vi "REACTOR_MODO MANUAL.vi"(5 "Modulo":u32, 7 "Secuencia":string[](array[string]), 8 "error in (no error)":errorcluster, 9 "ALICATS":T4=[["3", "NO", "M0000013", "Air", "10", "ln/mn", "0", "0"], ["4", "NO", "M0000014", "Air", "10", "ln/mn", "0", "0"], ["5", "NO", "M0000015", "Air", "10", "ln/mn", "0", "0"], ["6", "NO", "M0000016", "Air", "10", "ln/mn", "0", "0"], ["7", "NO", "M0000017", "Air", "10", "ln/mn", "0", "0"], ["8", "NO", "M0000018", "Air", "10", "ln/mn", "0", "0"]], 11 "Comms":T5={"Alicats"="ASRL6::INSTR", "Alic"=FALSE, "eValve"="ASRL6::INSTR", "eval"=FALSE, "Eurotherm"="ASRL6::INSTR", "euro"=FALSE, "Cell GAS"="ASRL6::INSTR", "cgas"=FALSE, "Cell H2S"="ASRL6::INSTR", "ch2s"=FALSE}) -> (0 "error out":errorcluster)   [LabVIEW 2017]
uses:
  REACTOR_DATOS.ctl
  REACTOR_COMUNICACIONES.ctl
  SERIAL ALICATS/__s_TablaAlicats.ctl
  SERIAL ALICATS/__Alicat SD_ReadingCluster.ctl
  EUROTHERM/TEG P116x2.ctl
  EUROTHERM/2xP116.ctl
  DISPLAY/Data Type.ctl
  DISPLAY/Display_Command Control.ctl
  REACTOR_MODO MANUAL.ctl
  FILE/File_Module Control.ctl
  TIMING/Timing_Module Control.ctl
  EUROTHERM/Eurotherm_New_Module.ctl
  REACTOR_CHANGE.ctl
  SERIAL RASP_PICO VALVE/kissia_rasPico Module.ctl
  REACTOR_GLOBALES.vi
panel:
  out "Fecha":string caption="asd"
  out "ERRORES_T":i32=5 caption="Elapsed Time (s)"
  out "VALVE":bool
  out "P116x2":T1
  out "ParsedReadingArray":T3[](array[typedef]) {"Total" format="%.2f"; "SetPoint" format="%.2f"; "Mass" format="%.2f"; "Volumetric" format="%.2f"; "Temperature" format="%.2f"; "Pressure" format="%.2f"}
  out "LEER ?":bool=TRUE
  in  "T.Wait Stability":bool
  in  "Mide Alicats":bool=TRUE
  in  "Mide Temperaturas":bool=TRUE
  in  "Muestreo(s)":dbl=1.0
  out "TIEMPO (m)":dbl
  out "Timestring":string
  out "idxModulo":u32
  out "Max_t(s)":dbl format="%.1f"
  out "Delta t(s)":dbl format="%.1f"
  out "Delta T(C)":dbl format="%.1f"
  out "TStable":bool
  out "Datos":T6 {"a FSET4" format="%.2g"; "a FSET3" format="%.2g"; "a FSET2" format="%.2g"; "a FSET1" format="%.2g"; "a FLUJO4" format="%.2g"; "a FLUJO2" format="%.2g"; "a FLUJO1" format="%.2g"; "a FLUJO3" format="%.2g"; "eVAL_5" format="%.2g"; "TEMP_TH" format="%.2g"; "SET_TH" format="%.2g"; "TEMP_TC" format="%.2g"; "SET_TC" format="%.2g"; "TIEMPO" format="%.2g"}
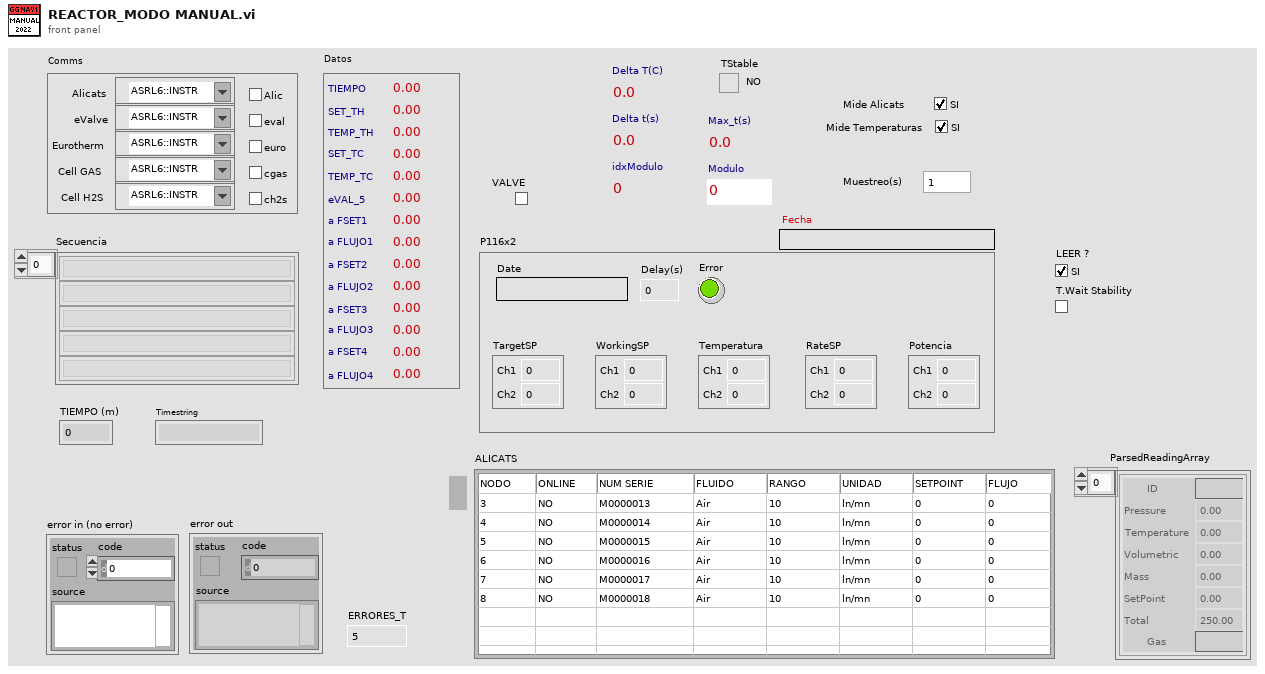
[diagram p1: front panel]
types:
  T1 = typedef "TEG P116x2.ctl" = cluster{"TargetSP":T2, "WorkingSP":T2, "Temperatura":T2, "Error":bool, "Date":string, "Delay(s)":dbl, "RateSP":T2, "Potencia":T2}
  T2 = typedef "2xP116.ctl" = cluster{"Ch1":dbl, "Ch2":dbl}
  T3 = typedef "__Alicat SD_ReadingCluster.ctl" = cluster{"ID":string, "Pressure":sgl, "Temperature":sgl, "Volumetric":sgl, "Mass":sgl, "SetPoint":sgl, "Gas":string, "Total":sgl}
  T4 = typedef "__s_TablaAlicats.ctl" = string[][]
  T5 = typedef "REACTOR_COMUNICACIONES.ctl" = cluster{"Alicats":refnum<visa-resource-name>, "Alic":bool, "eValve":refnum<visa-resource-name>, "eval":bool, "Eurotherm":refnum<visa-resource-name>, "euro":bool, "Cell GAS":refnum<visa-resource-name>, "cgas":bool, "Cell H2S":refnum<visa-resource-name>, "ch2s":bool}
  T6 = typedef "REACTOR_DATOS.ctl" = cluster{"TIEMPO":dbl, "SET_TH":dbl, "TEMP_TH":dbl, "SET_TC":dbl, "TEMP_TC":dbl, "eVAL_5":dbl, "a FSET1":dbl, "a FLUJO1":dbl, "a FSET2":dbl, "a FLUJO2":dbl, "a FSET3":dbl, "a FLUJO3":dbl, "a FSET4":dbl, "a FLUJO4":dbl}
  T7 = typedef "REACTOR_MODO MANUAL.ctl" = enum16{"INICIALIZAR", "LEER TIEMPO", "LEER TEMPERATURAS", "LEER ALICATS", "TEMPERATURAS ESTABLES ?", "GUARDAR DATOS", "WAIT NEXT", "HAY CAMBIOS ?", "FINALIZAR"}
  T8 = typedef "Data Type.ctl" = enum16{"Init FP", "En/Dis FP Ctls", "Update FP", "Upd Status", "Upd Seq"}
  T9 = typedef "Display_Command Control.ctl" = enum16{"Initialize", "Generate Event", "Shutdown"}
  T10 = typedef "File_Module Control.ctl" = enum16{"Initialize", "Save Head", "Save Data", "Shutdown"}
  T11 = typedef "Timing_Module Control.ctl" = enum16{"Initialize Time", "Check Time"}
  T12 = typedef "Eurotherm_New_Module.ctl" = enum16{"Initialize", "Write SP", "Read SP+PV", "Write Rate", "Set P", "Set I", "Set D", "Shutdown"}
  T13 = typedef "REACTOR_CHANGE.ctl" = enum16{"Default", "Continue", "Change Alicats", "Change Valve", "Change Calor", "Change Frio"}
  T14 = typedef "kissia_rasPico Module.ctl" = enum16{"Initialize", "Read Data", "Write Data", "Enable", "Disable", "Shutdown"}
  T15 = enum16{"Add 1", "Add 2", "Add 10", "Add 11", "Add 12", "Add 13"}[]
  T16 = cluster{"processVal":dbl, "targetSP":dbl, "workingSP":dbl, "workingOut":dbl}
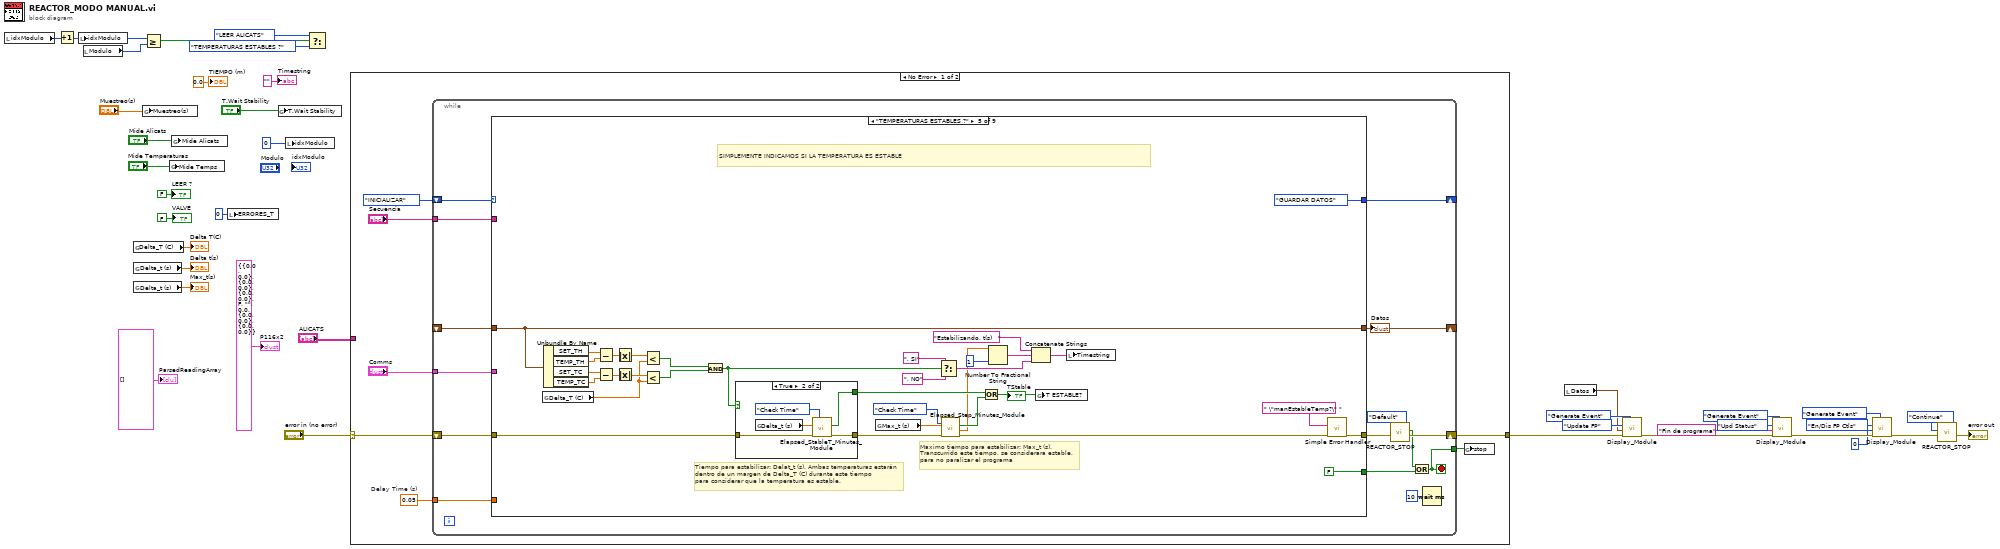
[diagram p0: block diagram]
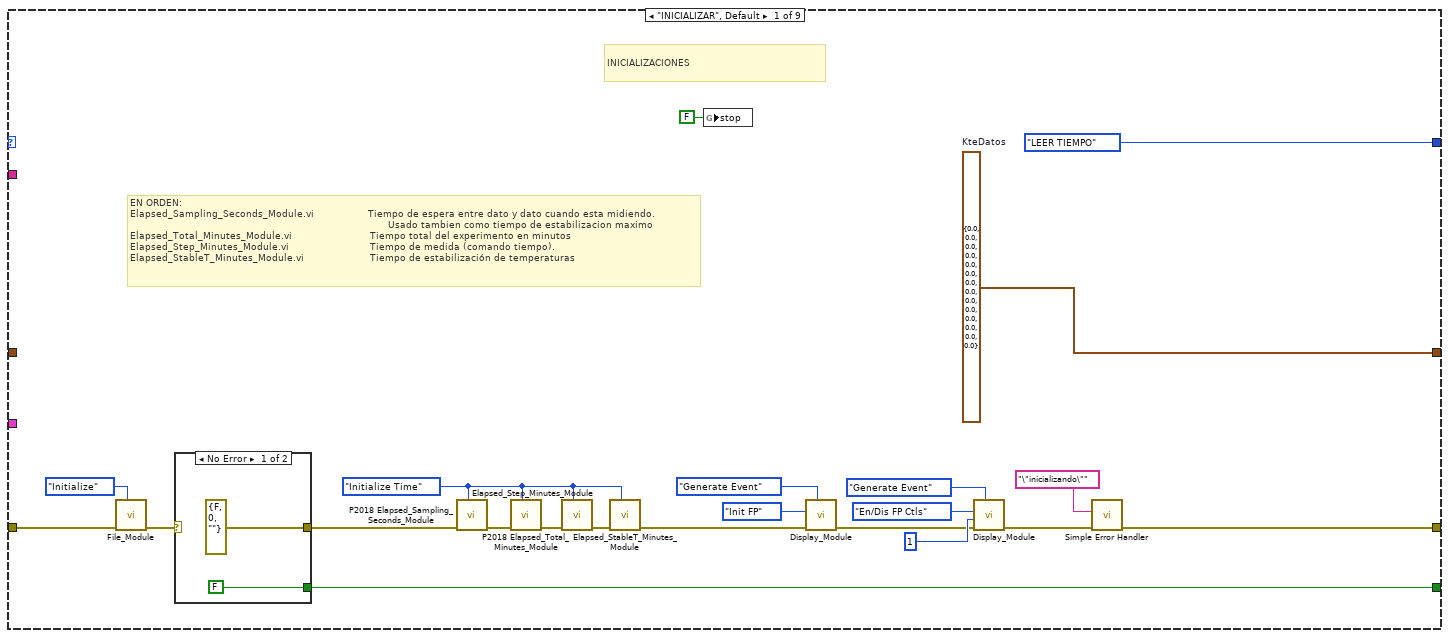
[diagram p2: hidden frame]
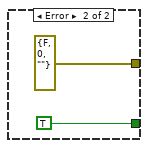
[diagram p3: hidden frame]
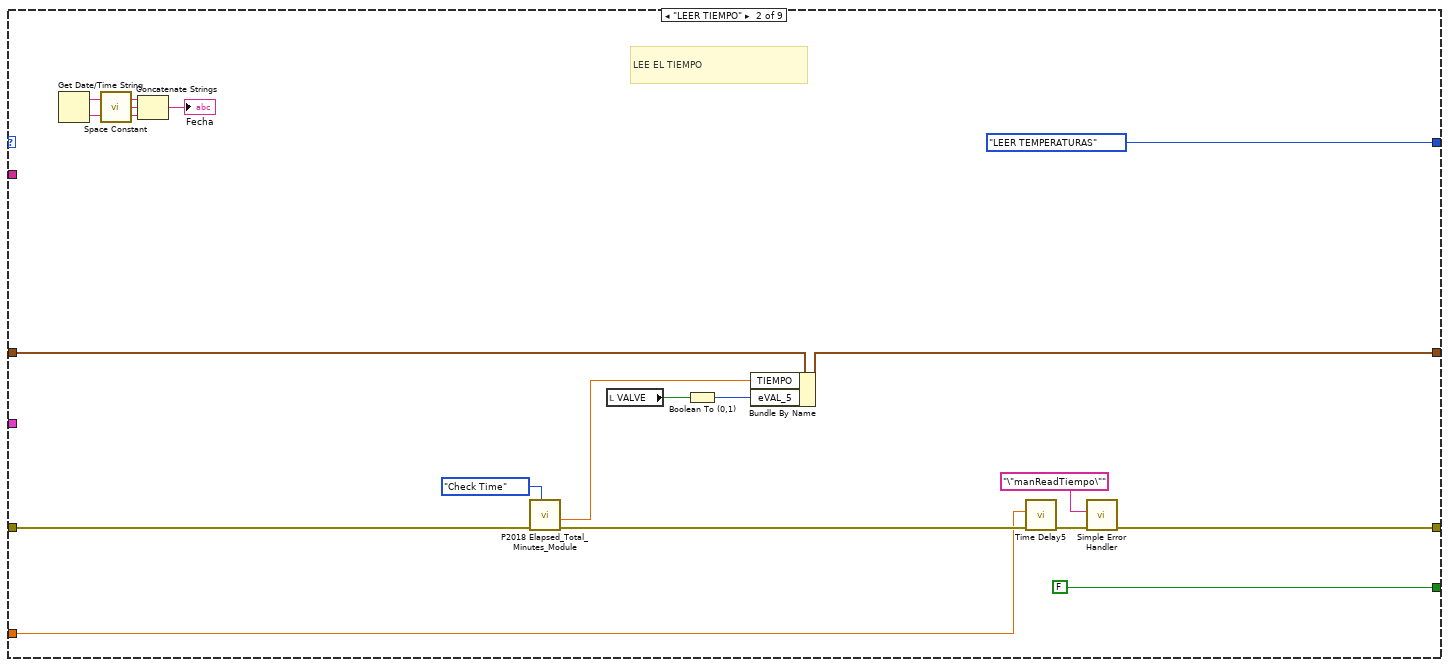
[diagram p4: hidden frame]
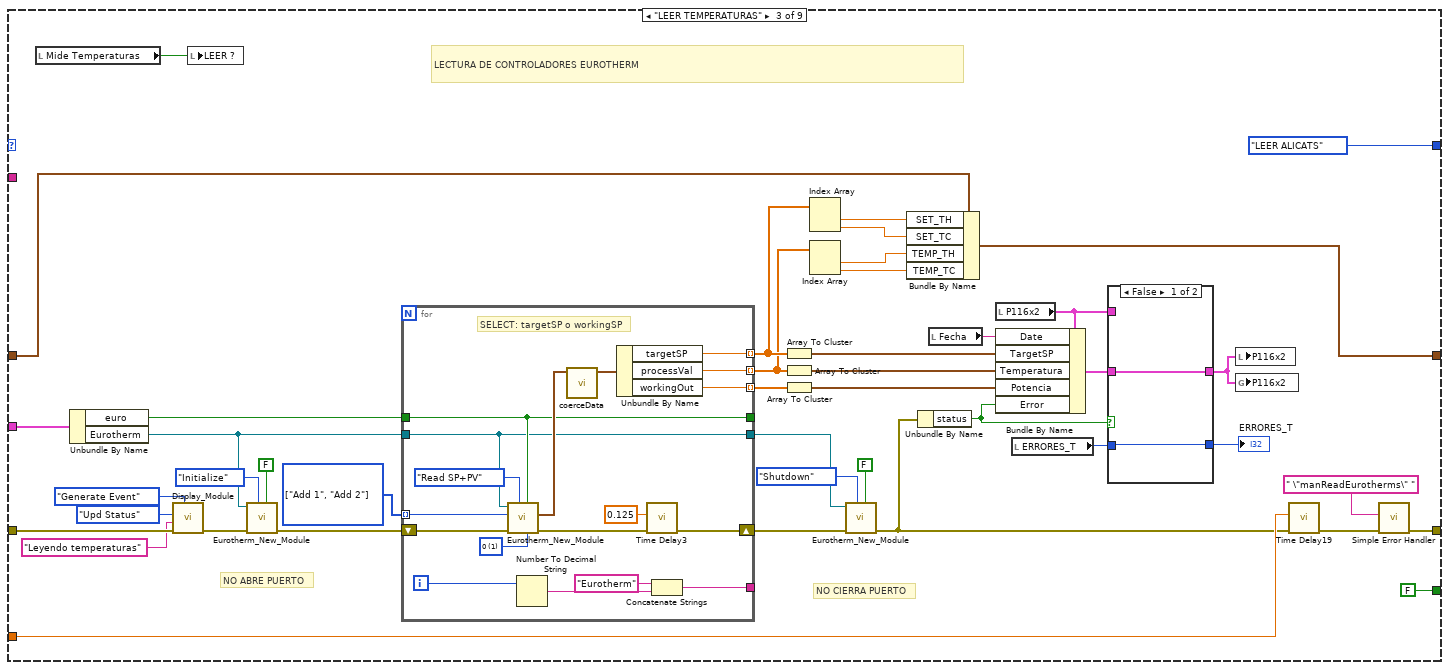
[diagram p5: hidden frame]
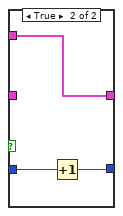
[diagram p6: hidden frame]
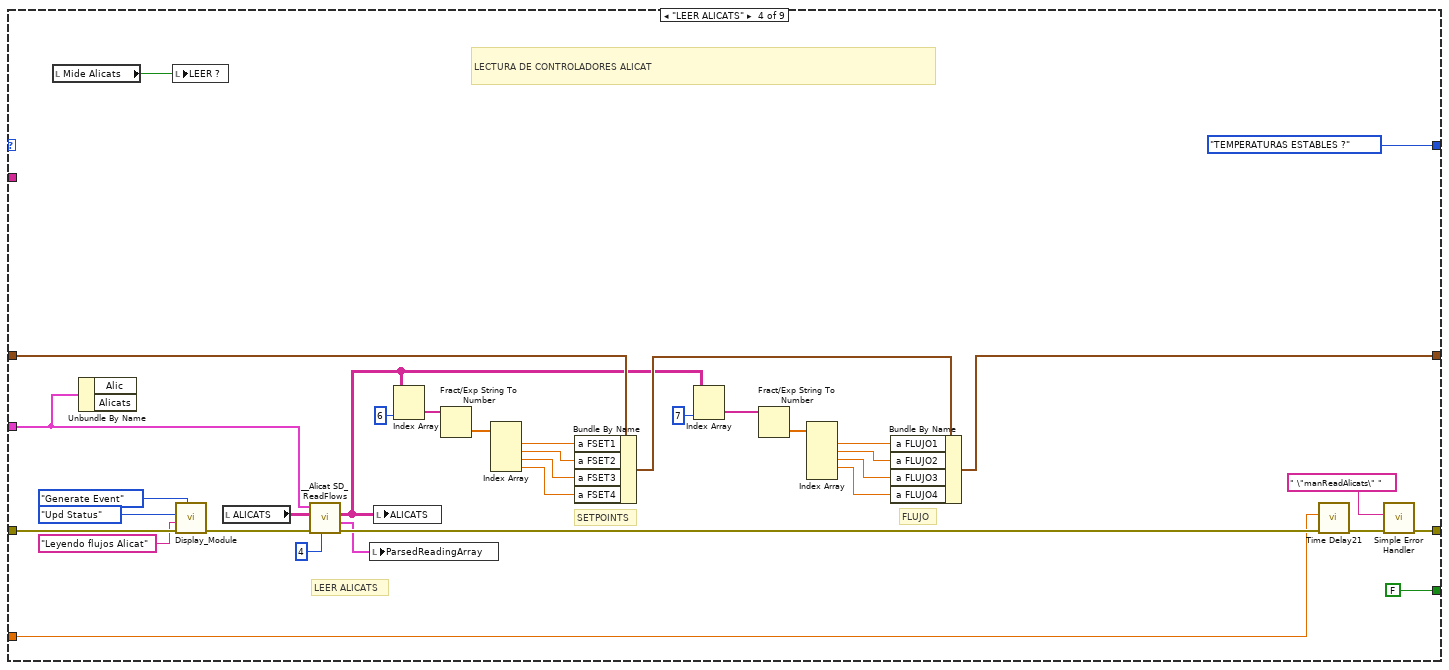
[diagram p7: hidden frame]
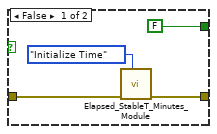
[diagram p8: hidden frame]
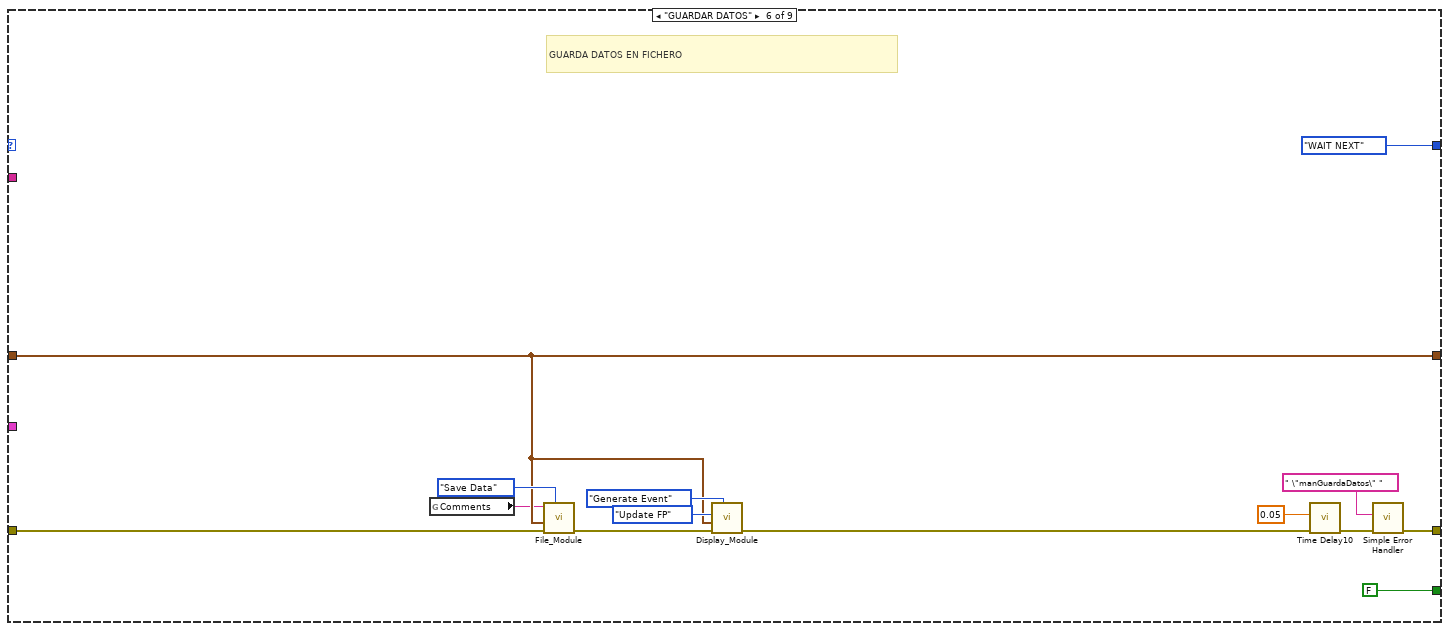
[diagram p9: hidden frame]
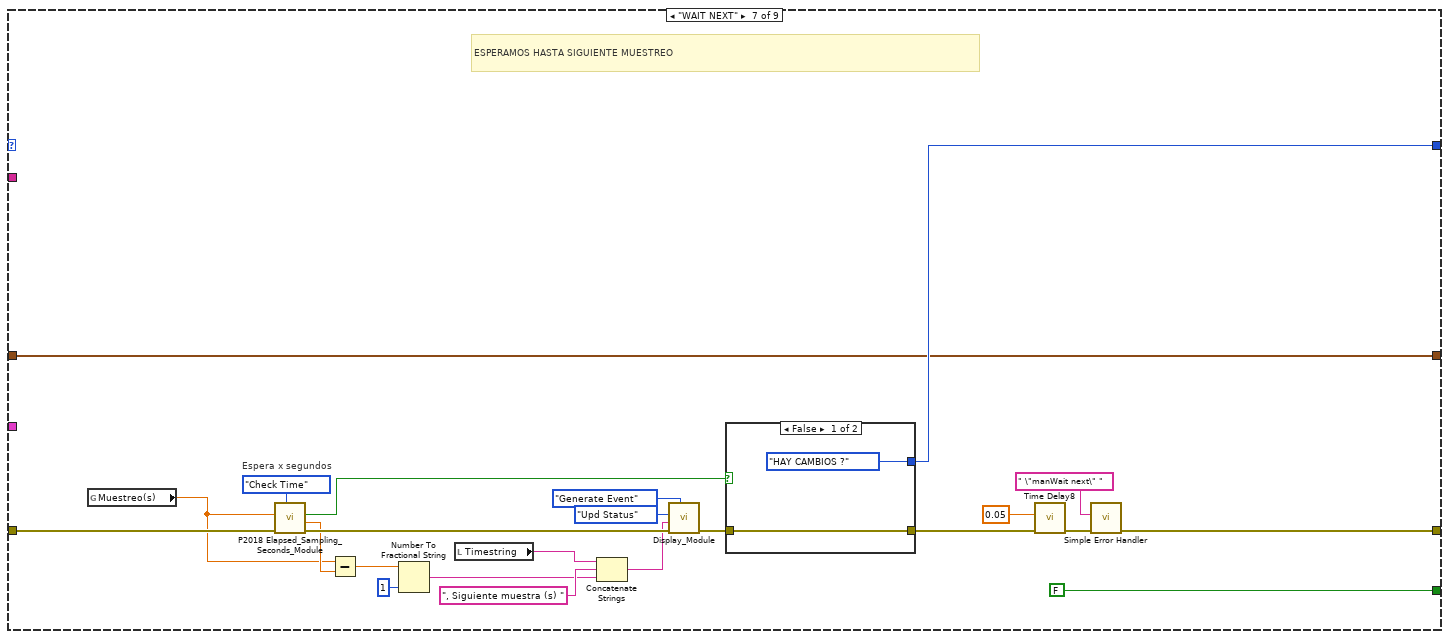
[diagram p10: hidden frame]
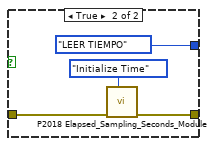
[diagram p11: hidden frame]
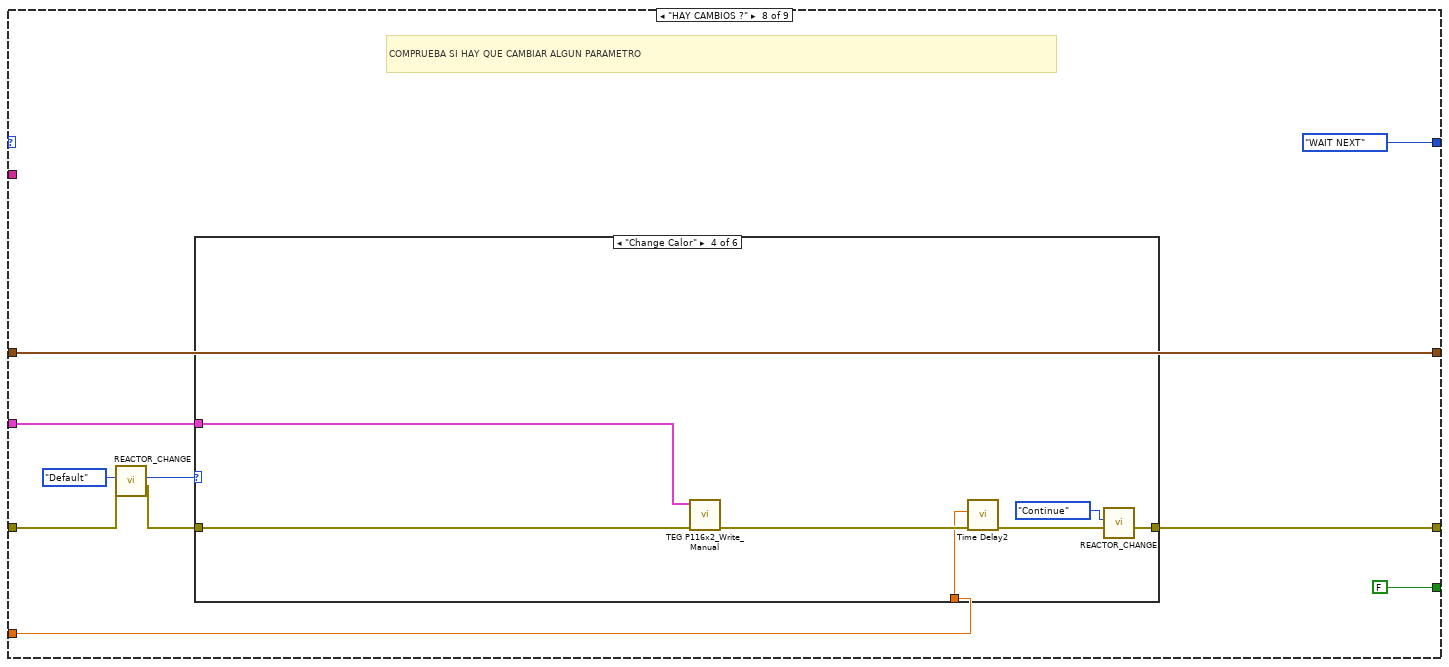
[diagram p12: hidden frame]
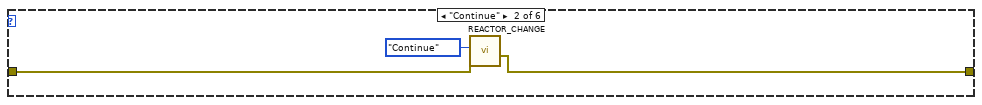
[diagram p14: hidden frame]
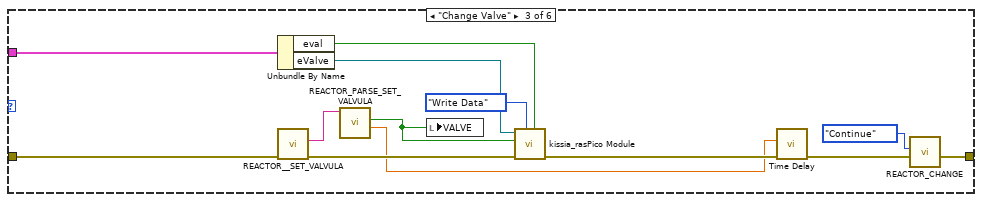
[diagram p15: hidden frame]
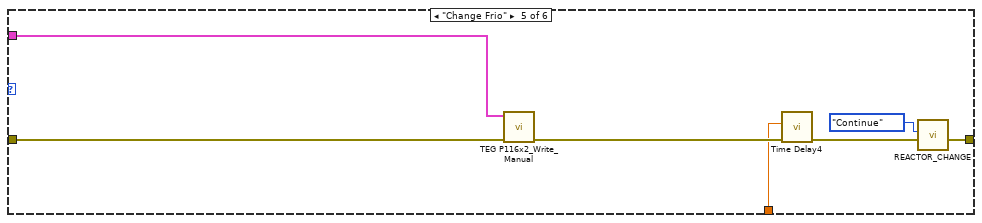
[diagram p16: hidden frame]
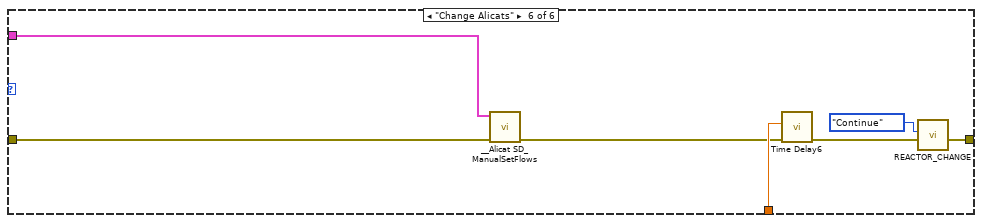
[diagram p17: hidden frame]
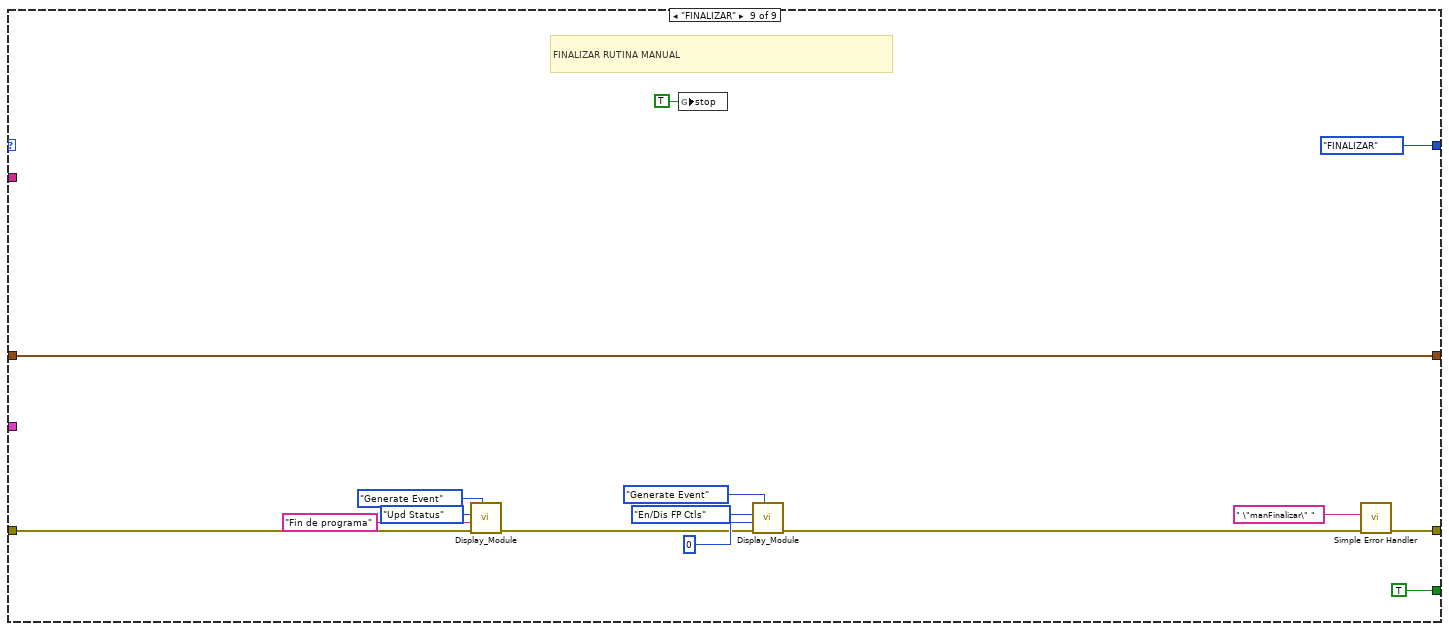
[diagram p18: hidden frame]
diagram:
  n1 = local read "idxModulo"() -> (w3:u32)
  n2 = Increment(x=w3) -> (x+1=w4:u32)
  n3 = local write "idxModulo"(w4) -> ()
  n4 = local read "Modulo"() -> (w6:u32)
  n5 = global read "REACTOR_GLOBALES.vi" "Delta_T (C)"() -> (→"Delta T(C)":dbl)
  n6 = global read "REACTOR_GLOBALES.vi" "Delta_t (s)"() -> (→"Delta t(s)":dbl)
  n7 = global read "REACTOR_GLOBALES.vi" "Delta_t (s)"() -> (→"Max_t(s)":dbl)
  n8 = global write "REACTOR_GLOBALES.vi" "Muestreo(s)"("Muestreo(s)") -> ()
  n9 = Greater Or Equal?(x=w4, y=w6) -> (x >= y?=w5:bool)
  n10 = global write "REACTOR_GLOBALES.vi" "Mide Temps"("Mide Temperaturas") -> ()
  n11 = global write "REACTOR_GLOBALES.vi" "Mide Alicats"("Mide Alicats") -> ()
  n12 = local write "ERRORES_T"(0 ("ERRORES_T")) -> ()
  n13 = global write "REACTOR_GLOBALES.vi" "T.Wait Stability"("T.Wait Stability") -> ()
  n14 = local write "idxModulo"(u32 0 ("MedidaModulo")) -> ()
  n15 = Select(t=REACTOR_MODO_MANUAL."LEER ALICATS" ("Command"), s=w5, f=REACTOR_MODO_MANUAL."TEMPERATURAS ESTABLES ?" ("Command")) -> ()  [unwired: 1 out]
  n16 = case shown="No Error" "error in (no error)" {
    selector: "error in (no error)" -> [w45 w354]
    tunnel: [w44 w354] -> w8
    tunnel: "ALICATS" -> [_ _]
    frame No Error {
      w40 = 0.05  # Delay Time (s)
      n17 = while {
        shift-right: [w56] -> _
        shift-left: REACTOR_MODO_MANUAL."INICIALIZAR" ("Command") -> [w57]
        shift-right: [w49] -> w44
        shift-left: w45 -> [w58]
        shift-right: [w53] -> _
        shift-left: _ -> [w55]
        tunnel: "Secuencia" -> [w54]
        tunnel: "Comms" -> [w52]
        tunnel: w40 -> [w51]
        tunnel: [w46] -> w39
        stop <- w46 stop-if-true
        n18 = case shown="\"TEMPERATURAS ESTABLES ?\"" w57 {
          tunnel: [w71 FALSE FALSE FALSE FALSE FALSE FALSE FALSE TRUE] -> w59
          tunnel: w58 -> [w81 w101 w144 w204 w208 w261 w278 w294 w349]
          tunnel: [w66 w98 w145 w202 w212 w253 w265 w296 w341] -> w50
          tunnel: [REACTOR_MODO_MANUAL."LEER TIEMPO" ("Command") REACTOR_MODO_MANUAL."LEER TEMPERATURAS" ("Command") REACTOR_MODO_MANUAL."LEER ALICATS" ("Command") REACTOR_MODO_MANUAL."TEMPERATURAS ESTABLES ?" ("Command") REACTOR_MODO_MANUAL."GUARDAR DATOS" ("Command") REACTOR_MODO_MANUAL."WAIT NEXT" ("Command") w281 REACTOR_MODO_MANUAL."WAIT NEXT" ("Command") REACTOR_MODO_MANUAL."FINALIZAR" ("Command")] -> w56
          tunnel: [w80 w102 w113 w176 w214 w255 w280 w298 w352] -> w53
          tunnel: w55 -> [_ w104 w114 w178 w214 w255 w280 w298 w352]
          tunnel: w54 -> [_ _ _ _ _ _ _ _ _]
          tunnel: w52 -> [_ _ w119 w173 _ _ _ w292 _]
          tunnel: w51 -> [_ w94 w139 w174 _ _ _ w291 _]
          frame "INICIALIZAR", Default {
            w63 = Timing_Module_Control."Initialize Time" ("Command")
            w80 = T6 {"TIEMPO"=0.0, "SET_TH"=0.0, "TEMP_TH"=0.0, "SET_TC"=0.0, "TEMP_TC"=0.0, "eVAL_5"=0.0, "a FSET1"=0.0, "a FLUJO1"=0.0, "a FSET2"=0.0, "a FLUJO2"=0.0, "a FSET3"=0.0, "a FLUJO3"=0.0, "a FSET4"=0.0, "a FLUJO4"=0.0}  # KteDatos
            # "INICIALIZACIONES"
            # "EN ORDEN:\nElapsed_Sampling_Seconds_Module.vi                  Tiempo de espera entre dato y dato cuando esta midiendo. \n                                                                                      Usado tambien como tiempo de estabilizacion maximo \nElapsed_Total_Minutes_Module.vi                          Tiempo total del experimento en minutos\nElapsed_Step_Minutes_Module.vi                           Tiempo de medida (comando tiempo). \nElapsed_StableT_Minutes_Module.vi                      Tiempo de estabilización de temperaturas"
            n19 = call "File_Module.vi"("Command"=File_Module_Control."Initialize", "error in (no error)"=w81) -> ("error out"=w73:errorcluster)  [unwired: 8 in, 1 out]
            n20 = case shown="No Error" w73 {
              tunnel: [errorcluster {"status"=FALSE, "code"=0, "source"=""} ("error out") errorcluster {"status"=FALSE, "code"=0, "source"=""} ("error out")] -> w72
              tunnel: [FALSE TRUE] -> w71
              frame No Error {
              }
              frame Error {
              }
            }
            n21 = call "P2018 Elapsed_Sampling_Seconds_Module.vi"("Command"=w63, "error in (no error)"=w72) -> ("error out"=w70:errorcluster)  [unwired: 7 in, 2 out]
            n22 = call "P2018 Elapsed_Total_Minutes_Module.vi"("Command"=w63, "error in (no error)"=w70) -> ("error out"=w69:errorcluster)  [unwired: 7 in, 2 out]
            n23 = call "Elapsed_Step_Minutes_Module.vi"("Command"=w63, "error in (no error)"=w69) -> ("error out"=w65:errorcluster)  [unwired: 7 in, 2 out]
            n24 = call "Elapsed_StableT_Minutes_Module.vi"("Command"=w63, "error in (no error)"=w65) -> ("error out"=w64:errorcluster)  [unwired: 7 in, 2 out]
            n25 = global write "REACTOR_GLOBALES.vi" "stop"(FALSE ("stop")) -> ()
            n26 = call "Display_Module.vi"("Command"=Display_Command_Control."Generate Event", "error in (no error)"=w64, "Data Type"=Data_Type."Init FP") -> ("error out"=w74:errorcluster)  [unwired: 8 in]
            n27 = call "Display_Module.vi"("Command"=Display_Command_Control."Generate Event", "error in (no error)"=w74, "Data"=1, "Data Type"=Data_Type."En/Dis FP Ctls") -> ("error out"=w67:errorcluster)  [unwired: 7 in]
            n28 = call <vilib>:"Simple Error Handler.vi"("error source (\" \")"="\"inicializando\"" ("error source (\" \")"), "error in (no error)"=w67) -> ("error out"=w66:errorcluster)  [unwired: 3 in, 4 out]
          }
          frame "LEER TIEMPO" {
            # "LEE EL TIEMPO"
            n29 = Get Date/Time String() -> (date string=w92:string, time string=w91:string)  [unwired: 3 in]
            n30 = call <vilib>:"Space Constant.vi"() -> ("String"=w90:string)
            n31 = Concatenate Strings(w92, w90, w91) -> (→"Fecha":string)
            n32 = call "P2018 Elapsed_Total_Minutes_Module.vi"("Command"=Timing_Module_Control."Check Time", "error in (no error)"=w101) -> ("error out"=w95:errorcluster, "Elapsed Out"=w97:dbl)  [unwired: 7 in, 1 out]
            n33 = local read "VALVE"() -> (w88:bool)
            n34 = Boolean To (0,1)(Boolean=w88) -> (0, 1=w87:i16)
            n35 = Bundle By Name(cluster=w104, "TIEMPO"=w97, "eVAL_5"=w87) -> (w102:T6)
            n36 = call "Time Delay5"("error in (no error)"=w95, "Delay Time (s)"=w94) -> ("error out"=w96:errorcluster)  [unwired: 9 in]
            n37 = call <vilib>:"Simple Error Handler.vi"("error source (\" \")"="\"manReadTiempo\"" ("error source (\" \")"), "error in (no error)"=w96) -> ("error out"=w98:errorcluster)  [unwired: 3 in, 4 out]
          }
          frame "LEER TEMPERATURAS" {
            w120 = T15 [enum."Add 1", enum."Add 2"] items=["Add 1", "Add 2", "Add 10", "Add 11", "Add 12", "Add 13"]
            # "LECTURA DE CONTROLADORES EUROTHERM"
            # "NO CIERRA PUERTO"
            # "NO ABRE PUERTO"
            n38 = local read "Mide Temperaturas"() -> (w137:bool)
            n39 = Unbundle By Name(w119) -> ("euro"=w133:bool, "Eurotherm"=w135:refnum<visa-resource-name>)
            n40 = call "Display_Module.vi"("Command"=Display_Command_Control."Generate Event", "error in (no error)"=w144, "Data"="Leyendo temperaturas", "Data Type"=Data_Type."Upd Status") -> ("error out"=w117:errorcluster)  [unwired: 7 in]
            n41 = local write "LEER ?"(w137) -> ()
            n42 = call "Eurotherm_New_Module.vi"("Eurotherm (T:Enable)"=FALSE, "Command"=Eurotherm_New_Module."Initialize", "error in (no error)"=w117, "VISA resource name"=w135) -> ("error out"=w132:errorcluster)  [unwired: 6 in, 1 out]
            n43 = for {
              tunnel: w120 -> [w153] mode=indexing
              tunnel: [w166] -> w112 mode=indexing
              tunnel: [w165] -> w111 mode=indexing
              shift-right: [w163] -> w134
              shift-left: w132 -> [w159]
              tunnel: w133 -> [w155]
              tunnel: [w168] -> _
              tunnel: [w164] -> w131 mode=indexing
              tunnel: [w155] -> _
              tunnel: w135 -> [w154]
              tunnel: [w154] -> w136
              i -> [w167]
              w156 = u16 1 items=["0"=1, "1"=10, "2"=100] ("Decimales")
              # "SELECT: targetSP o workingSP"
              n44 = call "Eurotherm_New_Module.vi"("Decimales"=w156, "Eurotherm (T:Enable)"=w155, "Command"=Eurotherm_New_Module."Read SP+PV", "error in (no error)"=w159, "Address"=w153, "VISA resource name"=w154) -> ("error out"=w160:errorcluster, "Eurotherm"=w157:T16)  [unwired: 4 in]
              n45 = Number To Decimal String(number=w167) -> (decimal integer string=w169:string)  [unwired: 1 in]
              n46 = call "coerceData.vi"("Eurotherm"=w157) -> ("Eurotherm 2"=w161:T16)  [unwired: 10 in]
              n47 = Unbundle By Name(w161) -> ("targetSP"=w166:dbl, "processVal"=w165:dbl, "workingOut"=w164:dbl)
              n48 = call "Time Delay3"("error in (no error)"=w160, "Delay Time (s)"=0.125) -> ("error out"=w163:errorcluster)  [unwired: 9 in]
              n49 = Concatenate Strings("Eurotherm" ("error source (\" \")"), w169) -> (w168:string)
            }
            n50 = Array To Cluster(array=w112) -> (cluster=w127:cluster{"[0]":dbl, "[1]":dbl})
            n51 = Array To Cluster(array=w111) -> (cluster=w126:cluster{"[0]":dbl, "[1]":dbl})
            n52 = Array To Cluster(array=w131) -> (cluster=w125:cluster{"[0]":dbl, "[1]":dbl})
            n53 = Index Array(array=w112) -> (element #1=w110:dbl, element #2=w109:dbl)  [unwired: 2 in]
            n54 = Index Array(array=w111) -> (element #1=w108:dbl, element #2=w107:dbl)  [unwired: 2 in]
            n55 = call "Eurotherm_New_Module.vi"("Eurotherm (T:Enable)"=FALSE, "Command"=Eurotherm_New_Module."Shutdown", "error in (no error)"=w134, "VISA resource name"=w136) -> ("error out"=w118:errorcluster)  [unwired: 6 in, 1 out]
            n56 = Bundle By Name(cluster=w114, "SET_TH"=w110, "SET_TC"=w109, "TEMP_TH"=w108, "TEMP_TC"=w107) -> (w113:T6)
            n57 = Unbundle By Name(w118) -> ("status"=w130:bool)
            n58 = local read "Fecha"() -> (w128:string)
            n59 = local read "P116x2"() -> (w115:T1)
            n60 = Bundle By Name(cluster=w115, "Date"=w128, "TargetSP"=w127, "Temperatura"=w126, "Potencia"=w125, "Error"=w130) -> (w129:T1)
            n61 = local read "ERRORES_T"() -> (w124:i32)
            n62 = case shown="False" w130 {
              tunnel: w129 -> [w149 _]
              tunnel: [w149 w150] -> w116
              tunnel: w115 -> [_ w150]
              tunnel: w124 -> [w148 w152]
              tunnel: [w148 w151] -> w123
              frame False {
              }
              frame True {
                n63 = Increment(x=w152) -> (x+1=w151:i32)
              }
            }
            "ERRORES_T" <- w123
            n64 = local write "P116x2"(w116) -> ()
            n65 = global write "REACTOR_GLOBALES.vi" "P116x2"(w116) -> ()
            n66 = call "Time Delay19"("error in (no error)"=w118, "Delay Time (s)"=w139) -> ("error out"=w140:errorcluster)  [unwired: 9 in]
            n67 = call <vilib>:"Simple Error Handler.vi"("error source (\" \")"=" \"manReadEurotherms\" " ("error source (\" \")"), "error in (no error)"=w140) -> ("error out"=w145:errorcluster)  [unwired: 3 in, 4 out]
          }
          frame "LEER ALICATS" {
            # "LECTURA DE CONTROLADORES ALICAT"
            # "FLUJO"
            # "SETPOINTS"
            # "LEER ALICATS"
            n68 = local read "Mide Alicats"() -> (w196:bool)
            n69 = Unbundle By Name(w173) -> ()  [unwired: 2 out]
            n70 = local write "LEER ?"(w196) -> ()
            n71 = call "Display_Module.vi"("Command"=Display_Command_Control."Generate Event", "error in (no error)"=w204, "Data"="Leyendo flujos Alicat", "Data Type"=Data_Type."Upd Status") -> ("error out"=w195:errorcluster)  [unwired: 7 in]
            n72 = local read "ALICATS"() -> (w172:T4)
            n73 = call "__Alicat SD_ReadFlows.vi"("Nodos"=4, "error in"=w195, "aDispositivos"=w172, "COMMS"=w173) -> ("error out"=w194:errorcluster, "ParsedReadingArray"=w175:T3[], "aDispositivos 2"=w171:T4)  [unwired: 5 in]
            n74 = local write "ParsedReadingArray"(w175) -> ()
            n75 = local write "ALICATS"(w171) -> ()
            n76 = Index Array(array=w171, index (col)=6 ("disabled index (col)")) -> (element=w190:string[])  [unwired: 1 in]
            n77 = Fract/Exp String To Number(string=w190) -> (number=w188:dbl[])  [unwired: 3 in, 1 out]
            n78 = Index Array(array=w188) -> (element #1=w186:dbl, element #2=w184:dbl, element #3=w183:dbl, element #4=w182:dbl)  [unwired: 4 in]
            n79 = Bundle By Name(cluster=w178, "a FSET1"=w186, "a FSET2"=w184, "a FSET3"=w183, "a FSET4"=w182) -> (w177:T6)
            n80 = Index Array(array=w171, index (col)=7 ("disabled index (col)")) -> (element=w189:string[])  [unwired: 1 in]
            n81 = Fract/Exp String To Number(string=w189) -> (number=w187:dbl[])  [unwired: 3 in, 1 out]
            n82 = Index Array(array=w187) -> (element #1=w185:dbl, element #2=w181:dbl, element #3=w180:dbl, element #4=w179:dbl)  [unwired: 5 in, 1 out]
            n83 = Bundle By Name(cluster=w177, "a FLUJO1"=w185, "a FLUJO2"=w181, "a FLUJO3"=w180, "a FLUJO4"=w179) -> (w176:T6)
            n84 = call "Time Delay21"("error in (no error)"=w194, "Delay Time (s)"=w174) -> ("error out"=w197:errorcluster)  [unwired: 9 in]
            n85 = call <vilib>:"Simple Error Handler.vi"("error source (\" \")"=" \"manReadAlicats\" " ("error source (\" \")"), "error in (no error)"=w197) -> ("error out"=w202:errorcluster)  [unwired: 3 in, 4 out]
          }
          frame "TEMPERATURAS ESTABLES ?" {
            # "SIMPLEMENTE INDICAMOS SI LA TEMPERATURA ES ESTABLE"
            # "Tiempo para estabilizar: Delat_t (s). Ambas temperaturas estarán \ndentro de un margen de Delta_T (C) durante este tiempo\npara considerar que la temperatura es estable."
            # "Maximo tiempo para estabilizar: Max_t (s). \nTranscurrido este tiempo, se considerara estable, \npara no paralizar el programa"
            n86 = global read "REACTOR_GLOBALES.vi" "Delta_T (C)"() -> (w229:dbl)
            n87 = Unbundle By Name(w214) -> ("SET_TH"=w237:dbl, "TEMP_TH"=w236:dbl, "SET_TC"=w235:dbl, "TEMP_TC"=w234:dbl)
            n88 = Subtract(x=w237, y=w236) -> (x-y=w233:dbl)
            n89 = Subtract(x=w235, y=w234) -> (x-y=w232:dbl)
            n90 = Absolute Value(x=w233) -> (abs(x)=w231:dbl)
            n91 = Absolute Value(x=w232) -> (abs(x)=w230:dbl)
            n92 = Less?(x=w231, y=w229) -> (x < y?=w227:bool)
            n93 = Less?(x=w230, y=w229) -> (x < y?=w228:bool)
            n94 = And(x=w227, y=w228) -> (x .and. y?=w216:bool)
            n95 = case shown="True" w216 {
              tunnel: w208 -> [w241 w246]
              tunnel: [w240 w245] -> w218
              tunnel: [FALSE ("TStable?") w244] -> w215
              frame False {
                n96 = call "Elapsed_StableT_Minutes_Module.vi"("Command"=Timing_Module_Control."Initialize Time", "error in (no error)"=w241) -> ("error out"=w240:errorcluster)  [unwired: 7 in, 2 out]
              }
              frame True {
                n97 = global read "REACTOR_GLOBALES.vi" "Delta_t (s)"() -> (w243:dbl)
                n98 = call "Elapsed_StableT_Minutes_Module.vi"("Command"=Timing_Module_Control."Check Time", "error in (no error)"=w246, "Time In"=w243) -> ("error out"=w245:errorcluster, "Time Elapsed"=w244:bool)  [unwired: 6 in, 1 out]
              }
            }
            n99 = global read "REACTOR_GLOBALES.vi" "Max_t (s)"() -> (w219:dbl)
            n100 = Select(t=", SI", s=w216, f=", NO") -> (s? t:f=w221:string)
            n101 = call "Elapsed_Step_Minutes_Module.vi"("Command"=Timing_Module_Control."Check Time", "error in (no error)"=w218, "Time In"=w219) -> ("error out"=w209:errorcluster, "Elapsed Out"=w211:dbl, "Time Elapsed"=w217:bool)  [unwired: 6 in]
            n102 = Or(x=w215, y=w217) -> (x .or. y?=w206:bool)
            "TStable" <- w206
            n103 = Number To Fractional String(number=w211, precision (6)=i16 1) -> (F-format string=w224:string)  [unwired: 2 in]
            n104 = Concatenate Strings("Estabilizando, t(s)   ", w224, w221) -> (w210:string)
            n105 = global write "REACTOR_GLOBALES.vi" "T ESTABLE?"(w206) -> ()
            n106 = local write "Timestring"(w210) -> ()
            n107 = call <vilib>:"Simple Error Handler.vi"("error source (\" \")"=" \"manEstableTemp?\" " ("error source (\" \")"), "error in (no error)"=w209) -> ("error out"=w212:errorcluster)  [unwired: 3 in, 4 out]
          }
          frame "GUARDAR DATOS" {
            # "GUARDA DATOS EN FICHERO"
            n108 = global read "REACTOR_GLOBALES.vi" "Comments"() -> (w252:string)
            n109 = call "File_Module.vi"("Command"=File_Module_Control."Save Data", "error in (no error)"=w261, "DATOS"=w255, "Comments"=w252) -> ("error out"=w256:errorcluster)  [unwired: 6 in, 1 out]
            n110 = call "Display_Module.vi"("Command"=Display_Command_Control."Generate Event", "error in (no error)"=w256, "Data"=w255, "Data Type"=Data_Type."Update FP") -> ("error out"=w249:errorcluster)  [unwired: 7 in]
            n111 = call "Time Delay10"("error in (no error)"=w249, "Delay Time (s)"=0.05) -> ("error out"=w248:errorcluster)  [unwired: 9 in]
            n112 = call <vilib>:"Simple Error Handler.vi"("error source (\" \")"=" \"manGuardaDatos\" " ("error source (\" \")"), "error in (no error)"=w248) -> ("error out"=w253:errorcluster)  [unwired: 3 in, 4 out]
          }
          frame "WAIT NEXT" {
            # "ESPERAMOS HASTA SIGUIENTE MUESTREO"
            # "Espera x segundos"
            n113 = global read "REACTOR_GLOBALES.vi" "Muestreo(s)"() -> (w262:dbl)
            n114 = call "P2018 Elapsed_Sampling_Seconds_Module.vi"("Command"=Timing_Module_Control."Check Time", "error in (no error)"=w278, "Time In"=w262) -> ("error out"=w277:errorcluster, "Elapsed Out"=w274:dbl, "Time Elapsed"=w275:bool)  [unwired: 6 in]
            n115 = Subtract(x=w262, y=w274) -> (x-y=w264:dbl)
            n116 = Number To Fractional String(number=w264, precision (6)=i16 1) -> (F-format string=w270:string)  [unwired: 2 in]
            n117 = local read "Timestring"() -> (w263:string)
            n118 = Concatenate Strings(w263, ", Siguiente muestra (s) ", w270) -> (w271:string)
            n119 = call "Display_Module.vi"("Command"=Display_Command_Control."Generate Event", "error in (no error)"=w277, "Data"=w271, "Data Type"=Data_Type."Upd Status") -> ("error out"=w276:errorcluster)  [unwired: 7 in]
            n120 = case shown="False" w275 {
              tunnel: [REACTOR_MODO_MANUAL."HAY CAMBIOS ?" ("Command") REACTOR_MODO_MANUAL."LEER TIEMPO" ("Command")] -> w281
              tunnel: w276 -> [w286 w289]
              tunnel: [w286 w288] -> w269
              frame False {
              }
              frame True {
                n121 = call "P2018 Elapsed_Sampling_Seconds_Module.vi"("Command"=Timing_Module_Control."Initialize Time", "error in (no error)"=w289) -> ("error out"=w288:errorcluster)  [unwired: 7 in, 2 out]
              }
            }
            n122 = call "Time Delay8"("error in (no error)"=w269, "Delay Time (s)"=0.05) -> ("error out"=w266:errorcluster)  [unwired: 9 in]
            n123 = call <vilib>:"Simple Error Handler.vi"("error source (\" \")"=" \"manWait next\" " ("error source (\" \")"), "error in (no error)"=w266) -> ("error out"=w265:errorcluster)  [unwired: 3 in, 4 out]
          }
          frame "HAY CAMBIOS ?" {
            # "COMPRUEBA SI HAY QUE CAMBIAR ALGUN PARAMETRO"
            n124 = call "REACTOR_CHANGE.vi"("error in (no error)"=w294, "Change"=REACTOR_CHANGE."Default") -> ("error out"=w293:errorcluster, "Change?"=w295:T13)  [unwired: 8 in]
            n125 = case shown="\"Change Calor\"" w295 {
              tunnel: w293 -> [w301 w303 w314 w320 w327 w334]
              tunnel: [w301 w302 w316 w323 w330 w337] -> w296
              tunnel: w292 -> [_ _ w309 w321 w328 w332]
              tunnel: w291 -> [_ _ _ w318 w325 w335]
              frame "Default", Default {
              }
              frame "Continue" {
                n126 = call "REACTOR_CHANGE.vi"("error in (no error)"=w303, "Change"=REACTOR_CHANGE."Continue") -> ("error out"=w302:errorcluster)  [unwired: 8 in, 1 out]
              }
              frame "Change Valve" {
                n127 = Unbundle By Name(w309) -> ("eval"=w306:bool, "eValve"=w308:refnum<visa-resource-name>)
                n128 = call "REACTOR__SET_VALVULA.vi"("error in (no error)"=w314) -> ("error out"=w313:errorcluster, "resulting string 1"=w315:string)  [unwired: 6 in, 1 out]
                n129 = call "REACTOR_PARSE_SET_VALVULA.vi"("String"=w315) -> ("Pausa (s)"=w310:dbl, "VALVULA 1"=w305:bool)  [unwired: 9 in]
                n130 = local write "VALVE"(w305) -> ()
                n131 = call "kissia_rasPico Module.vi"("Enable"=w306, "Command"=kissia_rasPico_Module."Write Data", "error in (no error)"=w313, "VALVE"=w305, "VISA resource name"=w308) -> ("error out"=w312:errorcluster)  [unwired: 3 in, 3 out]
                n132 = call "Time Delay"("error in (no error)"=w312, "Delay Time (s)"=w310) -> ("error out"=w311:errorcluster)  [unwired: 9 in]
                n133 = call "REACTOR_CHANGE.vi"("error in (no error)"=w311, "Change"=REACTOR_CHANGE."Continue") -> ("error out"=w316:errorcluster)  [unwired: 8 in, 1 out]
              }
              frame "Change Calor" {
                n134 = call "TEG P116x2_Write_Manual.vi"("error in (no error)"=w320, "Comunicaciones"=w321) -> ("error out"=w319:errorcluster)  [unwired: 7 in, 2 out]
                n135 = call "Time Delay2"("error in (no error)"=w319, "Delay Time (s)"=w318) -> ("error out"=w322:errorcluster)  [unwired: 9 in]
                n136 = call "REACTOR_CHANGE.vi"("error in (no error)"=w322, "Change"=REACTOR_CHANGE."Continue") -> ("error out"=w323:errorcluster)  [unwired: 8 in, 1 out]
              }
              frame "Change Frio" {
                n137 = call "TEG P116x2_Write_Manual.vi"("error in (no error)"=w327, "Comunicaciones"=w328) -> ("error out"=w326:errorcluster)  [unwired: 7 in, 2 out]
                n138 = call "Time Delay4"("error in (no error)"=w326, "Delay Time (s)"=w325) -> ("error out"=w329:errorcluster)  [unwired: 9 in]
                n139 = call "REACTOR_CHANGE.vi"("error in (no error)"=w329, "Change"=REACTOR_CHANGE."Continue") -> ("error out"=w330:errorcluster)  [unwired: 8 in, 1 out]
              }
              frame "Change Alicats" {
                n140 = call "__Alicat SD_ManualSetFlows.vi"("error in (no error)"=w334, "COMMS"=w332) -> ("error out"=w333:errorcluster)  [unwired: 6 in, 1 out]
                n141 = call "Time Delay6"("error in (no error)"=w333, "Delay Time (s)"=w335) -> ("error out"=w336:errorcluster)  [unwired: 9 in]
                n142 = call "REACTOR_CHANGE.vi"("error in (no error)"=w336, "Change"=REACTOR_CHANGE."Continue") -> ("error out"=w337:errorcluster)  [unwired: 8 in, 1 out]
              }
            }
          }
          frame "FINALIZAR" {
            # "FINALIZAR RUTINA MANUAL"
            n143 = call "Display_Module.vi"("Command"=Display_Command_Control."Generate Event", "error in (no error)"=w349, "Data"="Fin de programa", "Data Type"=Data_Type."Upd Status") -> ("error out"=w344:errorcluster)  [unwired: 7 in]
            n144 = global write "REACTOR_GLOBALES.vi" "stop"(TRUE ("stop")) -> ()
            n145 = call "Display_Module.vi"("Command"=Display_Command_Control."Generate Event", "error in (no error)"=w344, "Data"=0, "Data Type"=Data_Type."En/Dis FP Ctls") -> ("error out"=w342:errorcluster)  [unwired: 7 in]
            n146 = call <vilib>:"Simple Error Handler.vi"("error source (\" \")"=" \"manFinalizar\" " ("error source (\" \")"), "error in (no error)"=w342) -> ("error out"=w341:errorcluster)  [unwired: 3 in, 4 out]
          }
        }
        "Datos" <- w53
        n147 = call "REACTOR_STOP.vi"("error in (no error)"=w50, "Stop"=enum16{"Continue", "Stop", "Default"}."Default") -> ("error out"=w49:errorcluster, "Stop?"=w48:bool)  [unwired: 8 in]
        n148 = Or(x=w48, y=w59) -> (x .or. y?=w46:bool)
        n149 = Wait (ms)(milliseconds to wait=u32 10) -> ()  [unwired: 1 out]
      }
      n150 = global write "REACTOR_GLOBALES.vi" "stop"(w39) -> ()
    }
    frame Error {
    }
  }
  n151 = local read "Datos"() -> (w7:T6)
  n152 = call "Display_Module.vi"("Command"=Display_Command_Control."Generate Event", "error in (no error)"=w8, "Data"=w7, "Data Type"=Data_Type."Update FP") -> ("error out"=w9:errorcluster)  [unwired: 7 in]
  n153 = call "Display_Module.vi"("Command"=Display_Command_Control."Generate Event", "error in (no error)"=w9, "Data"="Fin de programa", "Data Type"=Data_Type."Upd Status") -> ("error out"=w37:errorcluster)  [unwired: 7 in]
  n154 = call "Display_Module.vi"("Command"=Display_Command_Control."Generate Event", "error in (no error)"=w37, "Data"=0, "Data Type"=Data_Type."En/Dis FP Ctls") -> ("error out"=w21:errorcluster)  [unwired: 7 in]
  n155 = call "REACTOR_STOP.vi"("error in (no error)"=w21, "Stop"=enum16{"Continue", "Stop", "Default"}."Continue") -> ("error out"=→"error out":errorcluster)  [unwired: 8 in, 1 out]
  "TIEMPO (m)" <- 0.0 ("TIEMPO (m)")
  "ParsedReadingArray" <- T3[] [] ("ParsedReadingArray")
  "P116x2" <- T1 {"TargetSP"={"Ch1"=0.0, "Ch2"=0.0}, "WorkingSP"={"Ch1"=0.0, "Ch2"=0.0}, "Temperatura"={"Ch1"=0.0, "Ch2"=0.0}, "Error"=FALSE, "Date"="", "Delay(s)"=0.0, "RateSP"={"Ch1"=0.0, "Ch2"=0.0}, "Potencia"={"Ch1"=0.0, "Ch2"=0.0}} ("P116x2")
  "VALVE" <- FALSE ("VALVE")
  "LEER ?" <- FALSE ("LEER ?")
  "Timestring" <- "" ("Timestring")
